vi "Tag_Details_PopUp.vi"(11 "Tag Ref in":refnum<data-value>) -> (3 "Tag Ref out":refnum<data-value>)   [LabVIEW 2020, in "Tag Watchlist.lvlib"]
doc: "Show details of selected tag"
uses:
  Tag Watchlist.lvlib
  Tag/Tag.lvclass
  Tag/Tag.lvclass/Tag.ctl
  Tag/Read Name.vi
  Tag/Read Value.vi
  Tag/Read Timestamp.vi
  Tag/Read Stale.vi
  Tag/Read Type.vi
  Tag/Read TypeString.vi
  cb32a538-1aa1-4039-9eea-9136e632c18e.vi
  Tag/Read ValChange.vi
  Tag/Get Property by Name.vi
  Tag/Read Property List.vi
  <vilib>/Utility/Data Type/Get Type Information.vi
  <vilib>/JDP Science/JSONtext/Variant to JSON Text.vi
  <vilib>/Utility/error.llb/Error Cluster From Error Code.vi
  Tag Engine.lvlib
  <vilib>/Utility/error.llb/whitespace.ctl
panel:
  out "dt":dbl format="%0.3f s"
  out "Stale":bool
  out "Timestamp":string
  out "Tag Name":string
  out "Data Type":string
  out "Value":string caption="Tag Value"
  out "Property Value":string
  in  "Property":string(combo)
  in  "Close":bool
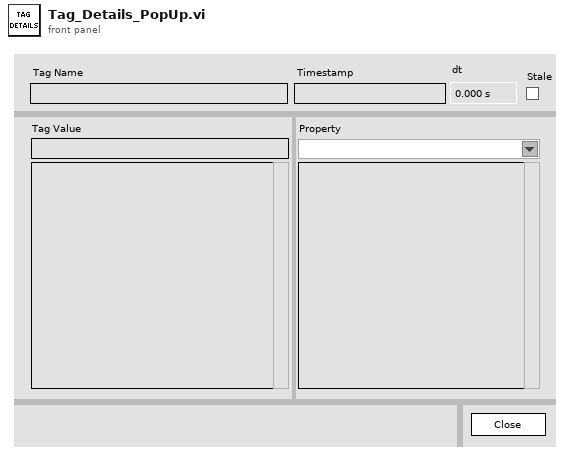
[diagram p1: front panel]
types:
  T1 = typedef "NI_Data Type.lvlib/Data Type.ctl" = enum8{"Invalid Type", "Void", "I8", "I16", "I32", "I64", "U8", "U16", "U32", "U64", "Single Float", "Double Float", "Extended Float", "Single Complex", "Double Complex", "Extended Complex", "Enum U8", "Enum U16", "Enum U32", "Enum U64", "Single Float With Unit", "Double Float With Unit", "Extended Float With Unit", "Single Complex with Unit", "Double Complex with Unit", "Extended Complex with Unit", "Boolean", "String", "Path", "Picture", "Tag", "Array", "Cluster", "Variant", "LV Variant", "Waveform", "Timestamp", "Digital Waveform", "Digital Data", "ExpressData", "Refnum", "External Data", "VI", "Poly VI", "LabVIEW Class Instance", "Fixed Point", "Set Collection", "Map Collection"}
  T2 = typedef "whitespace.ctl" = u16
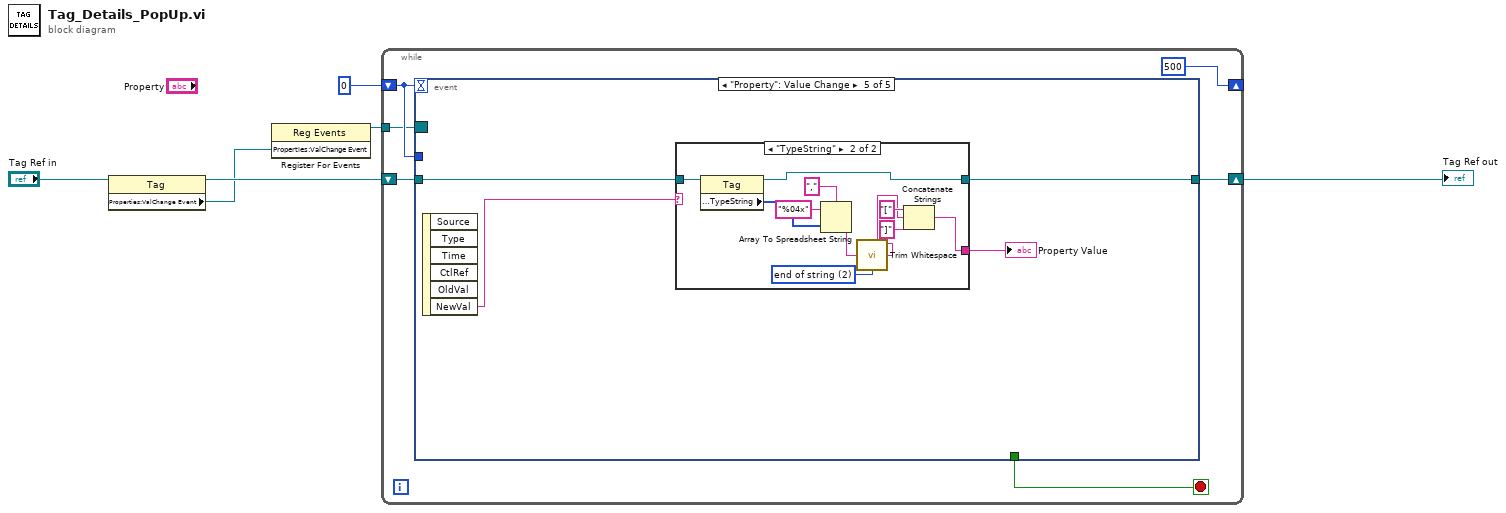
[diagram p0: block diagram]
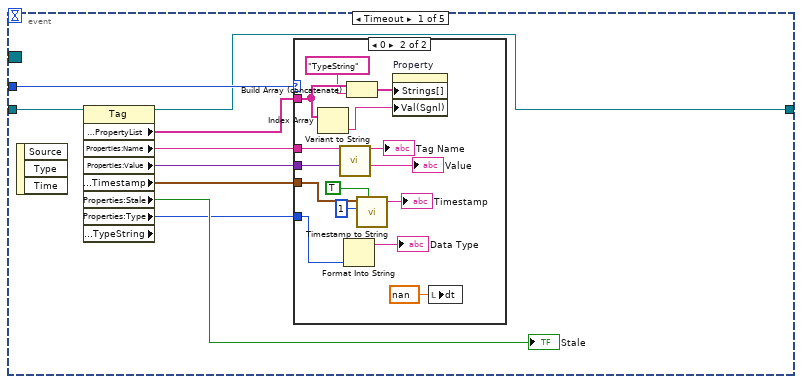
[diagram p2: hidden frame]
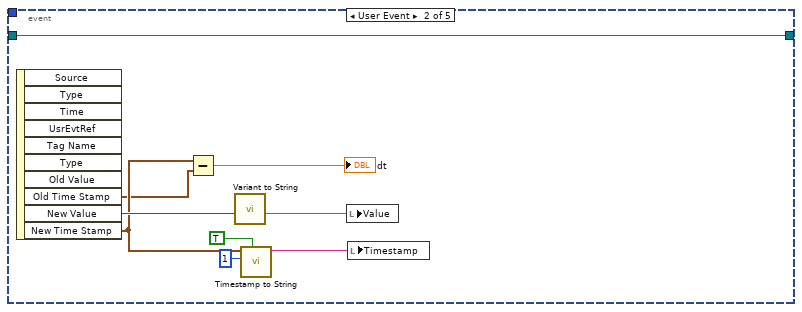
[diagram p4: hidden frame]
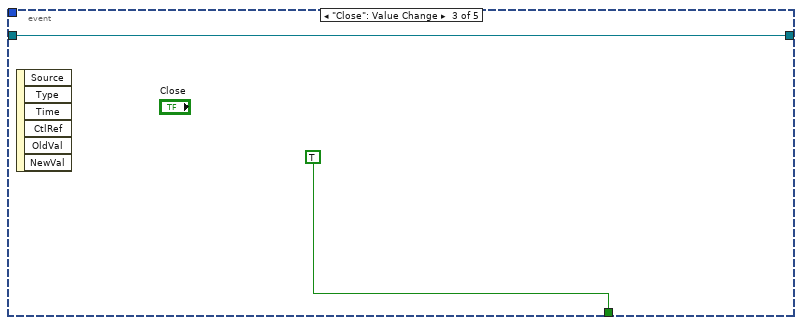
[diagram p5: hidden frame]
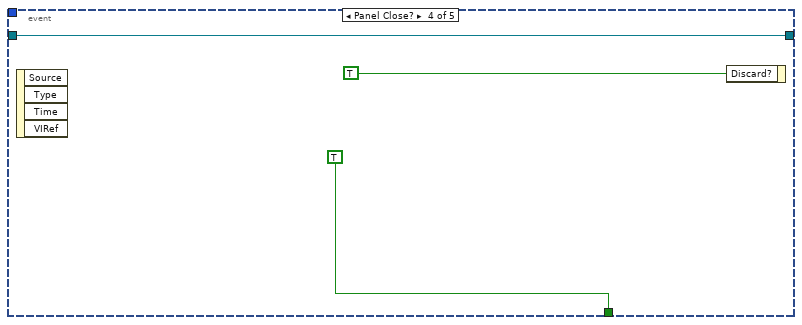
[diagram p6: hidden frame]
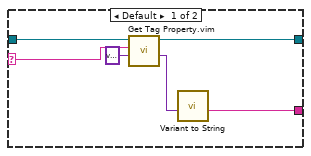
[diagram p7: hidden frame]
diagram:
  n1 = property class="Tag"(reference="Tag Ref in") -> (reference out=w3:refnum<data-value>, "Properties:ValChange Event"=w1:refnum<user-event>)  [unwired: 1 in, 1 out]
  n2 = register-events(w1) -> (reference out=w2:refnum<event-registration>)  [unwired: 2 in, 1 out]
  n3 = while {
    shift-right: [500] -> _
    shift-left: 0 -> [w8]
    tunnel: w2 -> [w7]
    shift-right: [w11] -> w6
    shift-left: w3 -> [w12]
    stop <- w10 stop-if-true
    n4 = event shown="[4] \"Property\": Value Change" {
      selector: w7 -> [_ _ _ _ _]
      dyn-events: _ -> [_ _ _ _ _]
      timeout: w8 -> [_ _ _ _ _]
      tunnel: w12 -> [w21 w43 w45 w47 w53]
      tunnel: [w17 w43 w45 w47 w52] -> w11
      tunnel: [_ _ TRUE TRUE _] -> w10
      tunnel: w8 -> [w18 _ _ _ _]
      event Timeout {
        n5 = event-data() -> ()  [unwired: 1 in, 3 out]
        n6 = property class="Tag" props=["Properties:PropertyList", "Properties:Name", "Properties:Value", "Properties:Timestamp", "Properties:Stale", "Properties:Type", "Properties:TypeString"](reference=w21) -> (reference out=w17:refnum<data-value>, "Properties:PropertyList"=w19:string[], "Properties:Name"=w15:string, "Properties:Value"=w14:variant, "Properties:Timestamp"=w13:timestamp, "Properties:Stale"=→"Stale":bool, "Properties:Type"=w16:T1)  [unwired: 1 in, 2 out]
        n7 = case shown="0" w18 {
          tunnel: w19 -> [_ w34]
          tunnel: w16 -> [_ w30]
          tunnel: w15 -> [_ w29]
          tunnel: w14 -> [_ w27]
          tunnel: w13 -> [_ w23]
          frame Default {
          }
          frame 0 {
            n8 = Index Array(array=w34) -> (element=w35:string)  [unwired: 1 in]
            n9 = call "Variant to String.vi"("Variant Value"=w27) -> ("String Value"=→"Value":string)  [unwired: 9 in, 1 out]
            n10 = Format Into String(w30) -> (resulting string=→"Data Type":string)  [unwired: 3 in, 1 out]
            n11 = Build Array (concatenate)(w34, "TypeString") -> (w32:string[])
            n12 = call "Timestamp to String.vi"("Include Date? (T)"=TRUE, "Precision (0)"=u8 1, "time stamp"=w23) -> ("date/time string"=→"Timestamp":string)  [unwired: 8 in]
            n13 = property on="Property" class="CmbBox"("Strings[]"=w32, "Val(Sgnl)"=w35) -> ()  [unwired: 2 in, 2 out]
            n14 = local write "dt"(nan ("dt")) -> ()
            "Tag Name" <- w29
          }
        }
      }
      event User Event {
        n15 = event-data() -> ("Old Time Stamp"=w37:timestamp, "New Value"=w40:variant, "New Time Stamp"=w38:timestamp)  [unwired: 1 in, 7 out]
        n16 = Subtract(x=w38, y=w37) -> (x-y=→"dt":dbl)
        n17 = call "Variant to String.vi"("Variant Value"=w40) -> ("String Value"=w44:string)  [unwired: 9 in, 1 out]
        n18 = call "Timestamp to String.vi"("Include Date? (T)"=TRUE, "Precision (0)"=u8 1, "time stamp"=w38) -> ("date/time string"=w39:string)  [unwired: 8 in]
        n19 = local write "Value"(w44) -> ()
        n20 = local write "Timestamp"(w39) -> ()
      }
      event "Close": Value Change {
        n21 = event-data() -> ()  [unwired: 1 in, 6 out]
      }
      event Panel Close? {
        n22 = event-data() -> ()  [unwired: 1 in, 4 out]
        n23 = event-data("Discard?"=TRUE) -> ()  [unwired: 1 in, 1 out]
      }
      event "Property": Value Change {
        n24 = event-data() -> ("NewVal"=w50:string)  [unwired: 1 in, 5 out]
        n25 = case shown="\"TypeString\"" w50 {
          selector: w50 -> [w54 _]
          tunnel: w53 -> [w58 w70]
          tunnel: [w57 w63] -> w52
          tunnel: [w55 w64] -> w51
          frame Default {
            n26 = call "Get Tag Property.vim"("Default (Void)"=variant, "PropertyName"=w54, "Tag Ref in"=w58) -> ("Value"=w56:variant, "Tag Ref out"=w57:refnum<data-value>)  [unwired: 5 in, 2 out]
            n27 = call "Variant to String.vi"("Variant Value"=w56) -> ("String Value"=w55:string)  [unwired: 9 in, 1 out]
          }
          frame "TypeString" {
            w61 = T2 2 items=["both", "start of string", "end of string"] ("location (both)")
            n28 = property class="Tag"(reference=w70) -> (reference out=w63:refnum<data-value>, "Properties:TypeString"=w69:i16[])  [unwired: 1 in, 1 out]
            n29 = Array To Spreadsheet String(delimiter (Tab)=",", array=w69, 3:"%04x" ("format string")) -> (spreadsheet string=w62:string)
            n30 = call <vilib>:"Trim Whitespace.vi"("string"=w62, "location (both)"=w61) -> ("trimmed string"=w60:string)
            n31 = Concatenate Strings("[" ("string"), w60, "]" ("string")) -> (w64:string)
          }
        }
        "Property Value" <- w51
      }
    }
  }
  "Tag Ref out" <- w6
